vi "SaveGpsRecordToKML.vi"(8 "error in (no error)":errorcluster caption="Fehler (Eingang, kein Fehler)", 10 "GPS_LogData":string) -> (0 "error out":errorcluster caption="Fehler (Ausgang)")   [LabVIEW 2017]
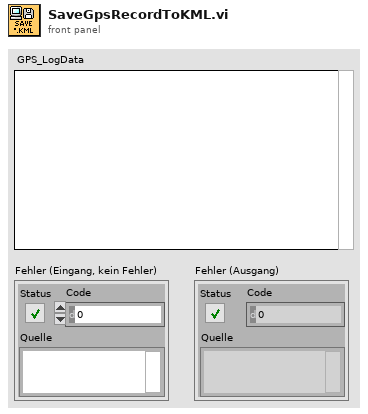
[diagram p1: front panel]
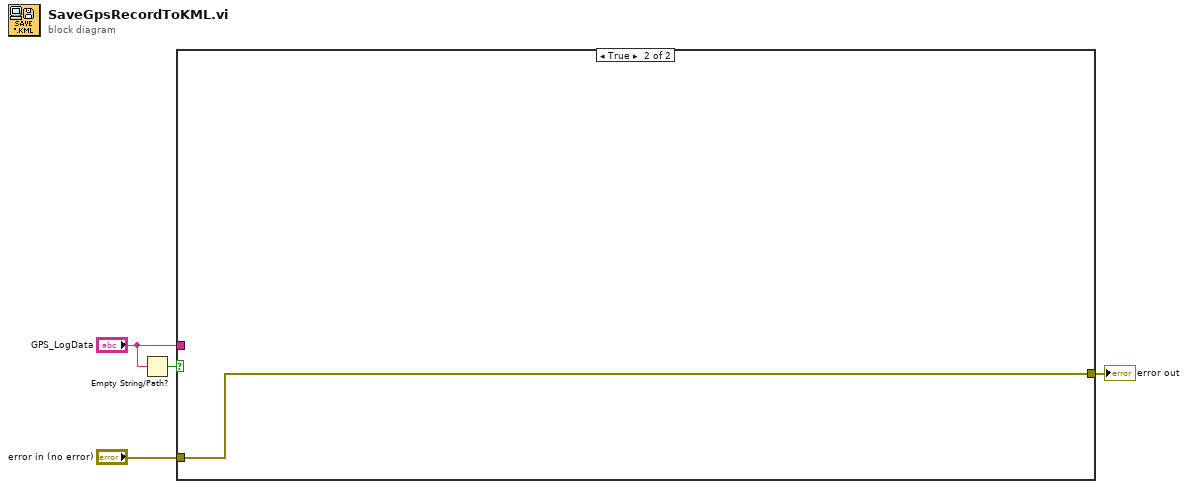
[diagram p0: block diagram]
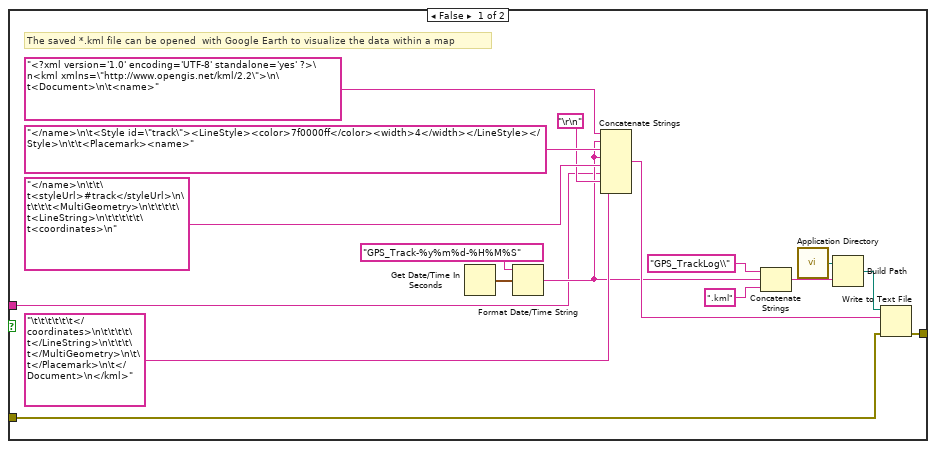
[diagram p2: hidden frame]
diagram:
  n1 = Empty String/Path?(string/path="GPS_LogData") -> (empty?=w1:bool)
  n2 = case shown="True" w1 {
    tunnel: [w11 w22] -> w4
    tunnel: "error in (no error)" -> [w10 w22]
    tunnel: "GPS_LogData" -> [w6 _]
    frame False {
      # "The saved *.kml file can be opened  with Google Earth to visualize the data within a map"
      n3 = Get Date/Time In Seconds() -> (seconds since 1Jan1904=w9:timestamp)
      n4 = Format Date/Time String(time format string (%c)="GPS_Track-%y%m%d-%H%M%S" ("Zeitformatierungs-String (%c)"), seconds (now)=w9) -> (date/time string=w7:string)  [unwired: 1 in]
      n5 = Concatenate Strings("<?xml version='1.0' encoding='UTF-8' standalone='yes' ?>\n<kml xmlns=\"http://www.opengis.net/kml/2.2\">\n\t<Document>\n\t<name>", w7, "</name>\n\t<Style id=\"track\"><LineStyle><color>7f0000ff</color><width>4</width></LineStyle></Style>\n\t\t<Placemark><name>", w7, "</name>\n\t\t\t<styleUrl>#track</styleUrl>\n\t\t\t\t<MultiGeometry>\n\t\t\t\t\t<LineString>\n\t\t\t\t\t\t<coordinates>\n", w6, "\r\n", "\t\t\t\t\t\t</coordinates>\n\t\t\t\t\t</LineString>\n\t\t\t\t</MultiGeometry>\n\t\t</Placemark>\n\t</Document>\n</kml>") -> (w14:string)
      n6 = Concatenate Strings("GPS_TrackLog\\" ("String"), w7, ".kml" ("String")) -> (w16:string)
      n7 = call <vilib>:"Application Directory.vi"() -> ("Application Directory"=w12:path)
      n8 = Build Path(base path=w12, name or relative path=w16) -> (appended path=w15:path)
      n9 = Write to Text File(file (use dialog)=w15, text=w14, error in=w10) -> (error out=w11:errorcluster)  [unwired: 1 in, 2 out]
    }
    frame True {
    }
  }
  "error out" <- w4
